vi "SIM Runge-Kutta (array).vi"(3 "Simulation data":T1={"continuous integrator"=enum."RK 1 (Euler)", "initial time"=0.1, "final time"=4.0, "step size"=600.0, "proposed step size"=1e-07, "max step size"=0.001, "min step size"=0.0, "discrete time step"=0.0, "max step ratio"=3.0, "Diag Eval Stage"=enum."Major Substep", "Substep Index"=0, "Timestep Index"=10.0, "simulation time"=0.0, "current timestep base"=0.01, "proposed step time"=0.0, "absolute tolerance"=0.0, "relative tolerance"=0.0, "step accepted?"=FALSE, "step complete?"=FALSE, "Halt?"=FALSE, "reset integrator?"=FALSE, "machine epsilon"=6.0, "min float"=0.0, "error"={"status"=FALSE, "code"=0, "source"=""}, "Method Order"=0, "Finished Late [i-1]"=FALSE, "Discrete step?"=FALSE, "NaN and Inf check?"=FALSE, "Final Timestep Index"=0.0, "(maj+disc)or(init)?"=FALSE, "Full Solver Reset"=TRUE, "Execution Mode"=enum."Simulate to Completion", "check vector sizes?"=FALSE, "solver handles zc?"=FALSE, "Simulation Registry"={"Current Idx"=0, "Node Tags"=[], "Node Headers"=[], "Node Data"=[], "Cont State data"={"inputs"=[], "outputs"=[], "reset"=[], "lower limits"=[], "upper limits"=[], "limit types"=[], "reset types"=[], "initial conditions"=[], "reset I.C."=[], "limited?"=[], "State Names"=[]}, "DiscreteInfo"={"tick period (sec)"=0.0, "time (ticks)"=0, "fire?"=[], "registry"={"period (sec)"=[], "skew (sec)"=[], "period (tick)"=[], "skew (tick)"=[]}, "discrete \nblocks?"=FALSE, "steps per tick"=0.0, "steps to tick"=0.0, "discrete \ntick?"=FALSE}, "Disc State data"={"Disc States"=[], "State Names"=[]}, "Registry Error"={"Error Block ID"=0, "code"=0}, "ZC Indices"=[]}, "variable step solver?"=FALSE, "First Substep?"=FALSE, "Continuous States?"=FALSE} {"min float" format="%.1e"; "proposed step size" format="%.1e"; "proposed step time" format="%.1e"; "max step ratio" format="%.1e"; "min step size" format="%.1e"; "machine epsilon" format="%.1e"; "discrete time step" format="%.1e"; "max step size" format="%.1e"; "current timestep base" format="%.1e"; "final time" format="%.1e"; "simulation time" format="%.1e"; "relative tolerance" format="%.1e"; "absolute tolerance" format="%.1e"; "Substep Index" format="%.1e"; "step size" format="%.1e"; "initial time" format="%.1e"}) -> (1 "Simulation data out":T1={"continuous integrator"=enum."RK 1 (Euler)", "initial time"=0.1, "final time"=4.0, "step size"=600.0, "proposed step size"=1e-07, "max step size"=0.001, "min step size"=0.0, "discrete time step"=0.0, "max step ratio"=3.0, "Diag Eval Stage"=enum."Major Substep", "Substep Index"=0, "Timestep Index"=10.0, "simulation time"=0.0, "current timestep base"=0.01, "proposed step time"=0.0, "absolute tolerance"=0.0, "relative tolerance"=0.0, "step accepted?"=FALSE, "step complete?"=FALSE, "Halt?"=FALSE, "reset integrator?"=FALSE, "machine epsilon"=6.0, "min float"=0.0, "error"={"status"=FALSE, "code"=0, "source"=""}, "Method Order"=0, "Finished Late [i-1]"=FALSE, "Discrete step?"=FALSE, "NaN and Inf check?"=FALSE, "Final Timestep Index"=0.0, "(maj+disc)or(init)?"=FALSE, "Full Solver Reset"=TRUE, "Execution Mode"=enum."Simulate to Completion", "check vector sizes?"=FALSE, "solver handles zc?"=FALSE, "Simulation Registry"={"Current Idx"=0, "Node Tags"=[], "Node Headers"=[], "Node Data"=[], "Cont State data"={"inputs"=[], "outputs"=[], "reset"=[], "lower limits"=[], "upper limits"=[], "limit types"=[], "reset types"=[], "initial conditions"=[], "reset I.C."=[], "limited?"=[], "State Names"=[]}, "DiscreteInfo"={"tick period (sec)"=0.0, "time (ticks)"=0, "fire?"=[], "registry"={"period (sec)"=[], "skew (sec)"=[], "period (tick)"=[], "skew (tick)"=[]}, "discrete \nblocks?"=FALSE, "steps per tick"=0.0, "steps to tick"=0.0, "discrete \ntick?"=FALSE}, "Disc State data"={"Disc States"=[], "State Names"=[]}, "Registry Error"={"Error Block ID"=0, "code"=0}, "ZC Indices"=[]}, "variable step solver?"=FALSE, "First Substep?"=FALSE, "Continuous States?"=FALSE} {"min float" format="%.1e"; "proposed step size" format="%.1e"; "proposed step time" format="%.1e"; "max step ratio" format="%.1e"; "min step size" format="%.1e"; "machine epsilon" format="%.1e"; "discrete time step" format="%.1e"; "max step size" format="%.1e"; "current timestep base" format="%.1e"; "final time" format="%.1e"; "simulation time" format="%.1e"; "relative tolerance" format="%.1e"; "absolute tolerance" format="%.1e"; "Substep Index" format="%.1e"; "step size" format="%.1e"; "initial time" format="%.1e"})   [LabVIEW 2014]
uses:
  SIM simulation data.ctl
  SIM integration method.ctl
  SIM diagram eval stage.ctl
  SIMSCR Execution Mode.ctl
  SIM Simulation Registry.ctl
  SIM Registry Node Header.ctl
  SIM Registry Node Record.ctl
  SIM trigger type.ctl
  SIM solver state data.ctl
  SIM limit type.ctl
  SIM discrete data.ctl
  SIM Discrete state data.ctl
  SIM Simulation Registry Error.ctl
  SIM limit signal (array).vi
panel:
  # "General Runge-Kutta integrator of order s.\n\nSolves the initial value problem \n\ny'(t) = f(t,y)\n\nby propogating the solution from y(t_n) to y(t_(n+1)), using the intermediate function evaluations k_i. The stepsize is defined as h = t_(n+1) - t_n.\n\nk_i = f( t_n + c_i h, y_n + h sum(j = 1 to s)(a_ij k_j) ) (1 <= i <= s)\n\ny_(n+1) = y_n + h sum(j = 1 to s)(a_(s-1)j k_j )\n\nNOTE This VI is paired with a time advancer that makes the simulation time appropriate for evaluating the k_i.\n\nNOTE This implementation assumes that c_0 = 0 and that\na_0j = 0 for a <= j <= s. The first row (all zeros) of the matrix a\nis omitted, and the last row of a stores the coefficients for the final output. Consequently, in the equation for k_i, a_ij should really read a_(i-1)j ."
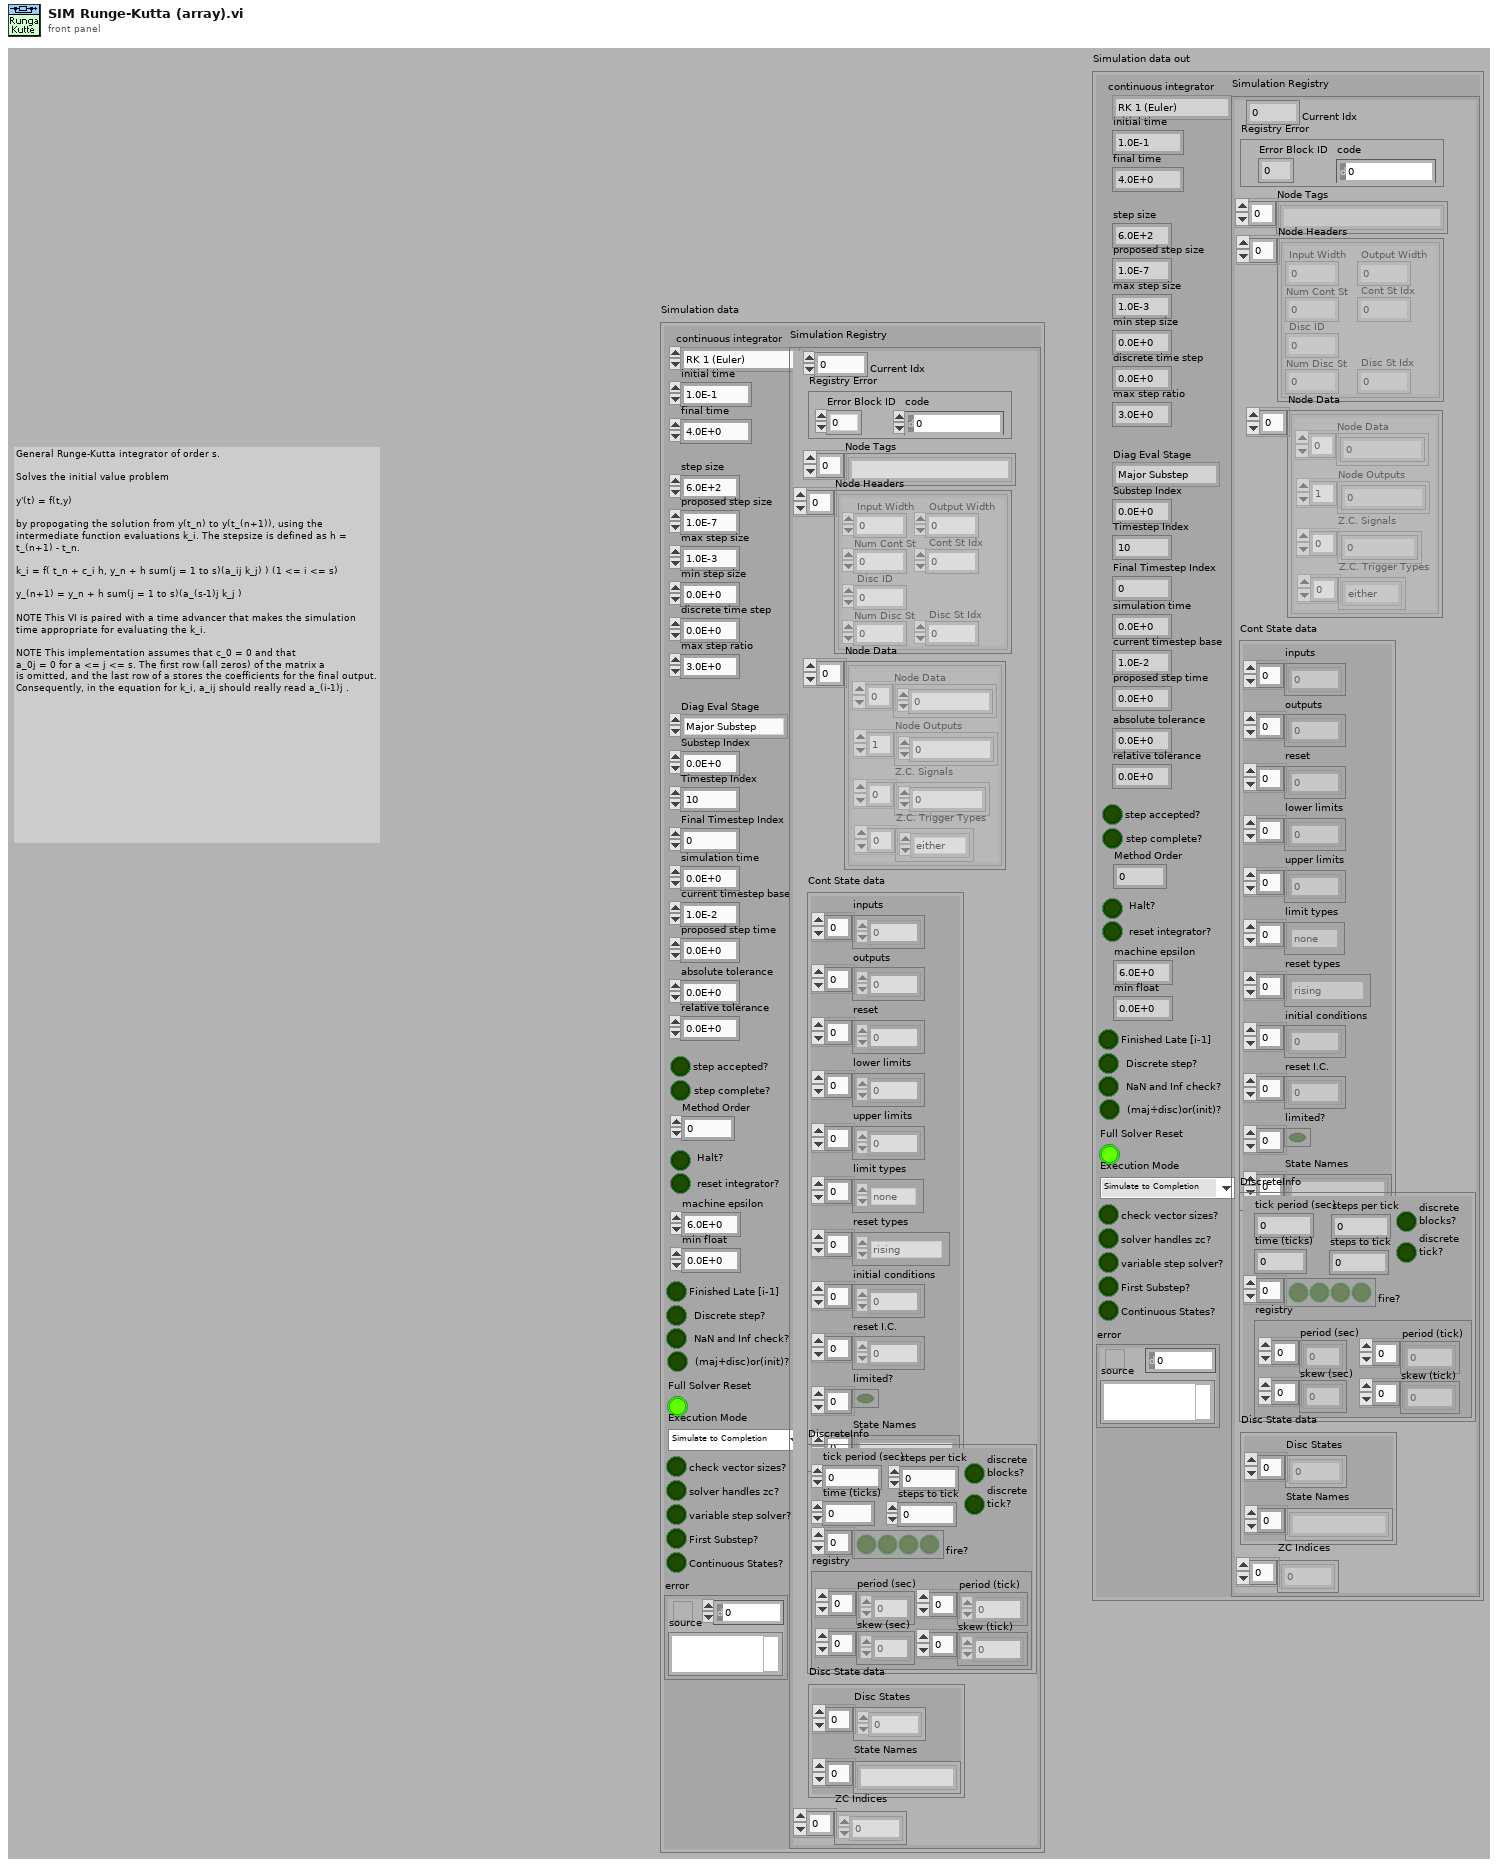
[diagram p1: front panel]
types:
  T1 = typedef "SIM simulation data.ctl" = cluster{"continuous integrator":T2, "initial time":dbl, "final time":dbl, "step size":dbl, "proposed step size":dbl, "max step size":dbl, "min step size":dbl, "discrete time step":dbl, "max step ratio":dbl, "Diag Eval Stage":T3, "Substep Index":i32, "Timestep Index":dbl, "simulation time":dbl, "current timestep base":dbl, "proposed step time":dbl, "absolute tolerance":dbl, "relative tolerance":dbl, "step accepted?":bool, "step complete?":bool, "Halt?":bool, "reset integrator?":bool, "machine epsilon":dbl, "min float":dbl, "error":errorcluster, "Method Order":u32, "Finished Late [i-1]":bool, "Discrete step?":bool, "NaN and Inf check?":bool, "Final Timestep Index":dbl, "(maj+disc)or(init)?":bool, "Full Solver Reset":bool, "Execution Mode":T4, "check vector sizes?":bool, "solver handles zc?":bool, "Simulation Registry":T5, "variable step solver?":bool, "First Substep?":bool, "Continuous States?":bool}
  T2 = typedef "SIM integration method.ctl" = enum16{"RK 1 (Euler)", "Linearizer", "State Query", "Trim Eval", "Adams", "RK 3", "RK 4", "RK 45", "BDF", "RK 2", "RK 23", "Rosenbrock", "Discrete States Only"}
  T3 = typedef "SIM diagram eval stage.ctl" = enum16{"Init", "Minor Substep", "Major Substep", "Final"}
  T4 = typedef "SIMSCR Execution Mode.ctl" = enum16{"Simulate to Completion", "Single Time-Step Simulation (Fixed Step Only)"}
  T5 = typedef "SIM Simulation Registry.ctl" = cluster{"Current Idx":i32, "Node Tags":string[], "Node Headers":T6[], "Node Data":T7[], "Cont State data":T9, "DiscreteInfo":T11, "Disc State data":T12, "Registry Error":T13, "ZC Indices":i32[]}
  T6 = typedef "SIM Registry Node Header.ctl" = cluster{"Input Width":i32, "Disc ID":i32, "Num Cont St":i32, "Cont St Idx":i32, "Num Disc St":i32, "Disc St Idx":i32, "Output Width":i32}
  T7 = typedef "SIM Registry Node Record.ctl" = cluster{"Node Data":dbl[], "Node Outputs":dbl[], "Z.C. Signals":dbl[], "Z.C. Trigger Types":T8[]}
  T8 = typedef "SIM trigger type.ctl" = enum16{"rising", "falling", "either", "none"}
  T9 = typedef "SIM solver state data.ctl" = cluster{"inputs":dbl[], "outputs":dbl[], "reset":dbl[], "lower limits":dbl[], "upper limits":dbl[], "limit types":T10[], "reset types":T8[], "initial conditions":dbl[], "reset I.C.":dbl[], "limited?":bool[], "State Names":string[]}
  T10 = typedef "SIM limit type.ctl" = enum16{"upper", "lower", "both", "none"}
  T11 = typedef "SIM discrete data.ctl" = cluster{"tick period (sec)":dbl, "time (ticks)":i32, "fire?":bool[], "registry":cluster{"period (sec)":dbl[], "skew (sec)":dbl[], "period (tick)":i32[], "skew (tick)":i32[]}, "discrete \nblocks?":bool, "steps per tick":dbl, "steps to tick":dbl, "discrete \ntick?":bool}
  T12 = typedef "SIM Discrete state data.ctl" = cluster{"Disc States":dbl[], "State Names":string[]}
  T13 = typedef "SIM Simulation Registry Error.ctl" = cluster{"Error Block ID":i32, "code":i32}
  T14 = typedef "SIM Runga-Kutte data - fixed step.ctl" = cluster{"weighting coefficients":dbl[][], "time step fractions":dbl[], "Number of sub steps":i32}
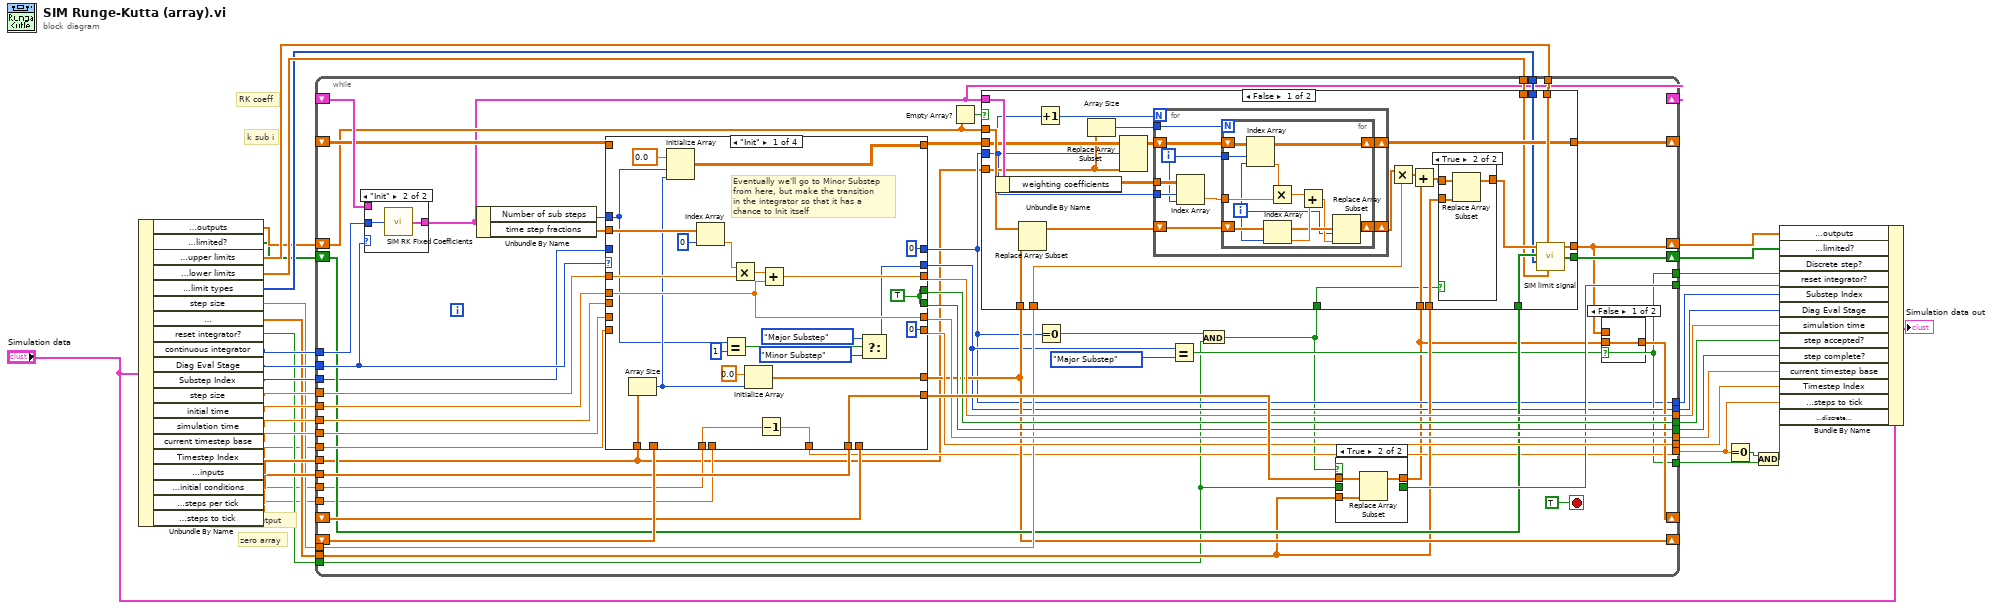
[diagram p0: block diagram]
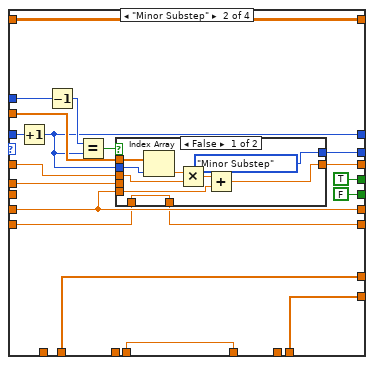
[diagram p6: hidden frame]
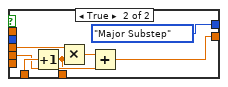
[diagram p7: hidden frame]
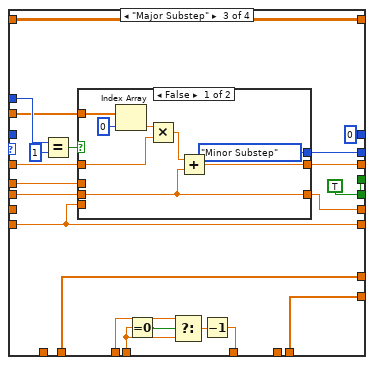
[diagram p8: hidden frame]
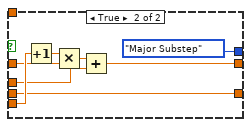
[diagram p9: hidden frame]
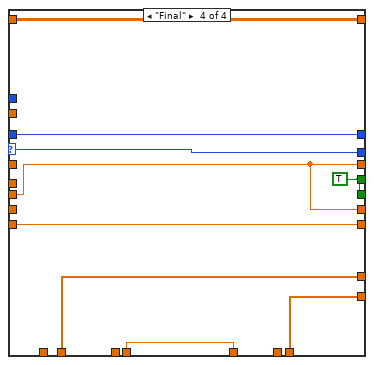
[diagram p10: hidden frame]
diagram:
  # "RK coeff"
  # "last major output"
  # "k sub i"
  # "zero array"
  n1 = Unbundle By Name("Simulation data") -> ("Simulation Registry.Cont State data.outputs"=w12:dbl[], "Simulation Registry.Cont State data.limited?"=w11:bool[], "Simulation Registry.Cont State data.upper limits"=w25:dbl[], "Simulation Registry.Cont State data.lower limits"=w24:dbl[], "Simulation Registry.Cont State data.limit types"=w23:T10[], "step size"=w16:dbl, "Simulation Registry.Cont State data.reset I.C."=w15:dbl[], "reset integrator?"=w13:bool, "continuous integrator"=w35:T2, "Diag Eval Stage"=w34:T3, "Substep Index"=w33:i32, "step size"=w32:dbl, "initial time"=w31:dbl, "simulation time"=w30:dbl, "current timestep base"=w29:dbl, "Timestep Index"=w9:dbl, "Simulation Registry.Cont State data.inputs"=w28:dbl[], "Simulation Registry.Cont State data.initial conditions"=w27:dbl[], "Simulation Registry.DiscreteInfo.steps per tick"=w6:dbl, "Simulation Registry.DiscreteInfo.steps to tick"=w5:dbl)
  n2 = while {
    shift-right: [w60] -> _
    shift-left: _ -> [w84]
    tunnel: w23 -> [w48]
    tunnel: w24 -> [w58]
    tunnel: w25 -> [w63]
    shift-right: [w55] -> _
    shift-left: _ -> [w81]
    shift-right: [w59] -> _
    shift-left: _ -> [w83]
    tunnel: [w49] -> w8
    shift-right: [w38] -> _
    shift-left: _ -> [w87]
    tunnel: w35 -> [w78]
    tunnel: w34 -> [w77]
    tunnel: w33 -> [w51]
    tunnel: w32 -> [w76]
    tunnel: w31 -> [w75]
    tunnel: w30 -> [w74]
    tunnel: w29 -> [w73]
    tunnel: w9 -> [w72]
    tunnel: w28 -> [w44]
    tunnel: w27 -> [w71]
    tunnel: [w47] -> w22
    tunnel: [w50] -> w21
    tunnel: [w70] -> w20
    tunnel: [w69] -> w19
    tunnel: [w68] -> w18
    tunnel: [w67] -> w17
    tunnel: [w66] -> w7
    tunnel: w16 -> [w65]
    tunnel: w15 -> [w57]
    tunnel: w13 -> [w42]
    tunnel: [w64] -> w14
    shift-right: [w56] -> w37
    shift-left: w12 -> [w40]
    shift-right: [w62] -> w10
    shift-left: w11 -> [w61]
    tunnel: w6 -> [w53]
    tunnel: w5 -> [w54]
    tunnel: [w52] -> w4
    tunnel: [w49] -> w2
    stop <- TRUE stop-if-true
    n3 = case shown="\"Init\"" w77 {
      tunnel: [w253 w255] -> w38
      tunnel: w87 -> [w253 _]
      tunnel: w78 -> [_ w254]
      frame Default {
      }
      frame "Init" {
        n4 = call "SIM RK Fixed Coefficients.vi"("continuous integrator"=w254) -> ("Runga-Kutte data out"=w255:T14)
      }
    }
    n5 = Unbundle By Name(w38) -> ("Number of sub steps"=w86:i32, "time step fractions"=w85:dbl[])
    n6 = case shown="\"Init\"" w77 {
      selector: w77 -> [_ _ _ w250]
      tunnel: w76 -> [w168 w183 w225 _]
      tunnel: [w165 w188 w223 w249] -> w67
      tunnel: w73 -> [_ w188 _ _]
      tunnel: w85 -> [w171 w190 w219 _]
      tunnel: [w166 w189 w220 w249] -> w70
      tunnel: w72 -> [_ w174 w213 w247]
      tunnel: w86 -> [w149 w187 w227 _]
      tunnel: [w152 w180 w217 w250] -> w50
      tunnel: w75 -> [w165 w179 w224 _]
      tunnel: [0 ("Timestep Index") w173 w213 w247] -> w66
      tunnel: w74 -> [_ _ w221 w249]
      tunnel: [w150 TRUE w207 w248] -> w69
      tunnel: [w150 FALSE w207 w248] -> w68
      tunnel: w51 -> [_ w182 _ w252]
      tunnel: [0 w178 0 ("Substep Index") w252] -> w47
      tunnel: w44 -> [w162 _ _ _]
      tunnel: [w158 w176 w216 w251] -> w46
      tunnel: w84 -> [_ w176 w216 w251]
      tunnel: [w157 w177 w215 w245] -> w59
      tunnel: w83 -> [_ w177 w215 w245]
      tunnel: w81 -> [_ w175 w214 w246]
      tunnel: [w151 w175 w214 w246] -> w80
      tunnel: w71 -> [w151 _ _ _]
      tunnel: w54 -> [_ w172 w209 w244]
      tunnel: w53 -> [w147 _ w210 _]
      tunnel: [w148 w172 w208 w244] -> w52
      frame "Init" {
        w150 = TRUE
        # "Eventually we'll go to Minor Substep from here, but make the transition in the integrator so that it has a chance to Init itself"
        n7 = Array Size(array=w162) -> (size(s)=w159:i32)
        n8 = Initialize Array(0.0 ("element"), w149, w159) -> (w158:dbl[][])
        n9 = Index Array(array=w171, index=0) -> (element=w169:dbl)
        n10 = Equal?(x=w149, y=1) -> (x = y?=w153:bool)
        n11 = Multiply(x=w169, y=w168) -> (x*y=w167:dbl)
        n12 = Initialize Array(0.0 ("element"), w159) -> (w157:dbl[])
        n13 = Decrement(x=w147) -> (x-1=w148:dbl)
        n14 = Add(x=w167, y=w165) -> (x+y=w166:dbl)
        n15 = Select(t=SIM_diagram_eval_stage."Major Substep", s=w153, f=SIM_diagram_eval_stage."Minor Substep" ("Diagram Eval Stage")) -> (s? t:f=w152:T3)
      }
      frame "Minor Substep" {
        n16 = Increment(x=w182) -> (x+1=w178:i32)
        n17 = Decrement(x=w187) -> (x-1=w186:i32)
        n18 = Equal?(x=w186, y=w178) -> (x = y?=w181:bool)
        n19 = case shown="False" w181 {
          tunnel: w190 -> [w199 _]
          tunnel: [w196 w201] -> w189
          tunnel: w188 -> [w195 _]
          tunnel: w183 -> [w194 w204]
          tunnel: w178 -> [w193 _]
          tunnel: [SIM_diagram_eval_stage."Minor Substep" ("f") SIM_diagram_eval_stage."Major Substep" ("Diagram Eval Stage")] -> w180
          tunnel: w174 -> [w191 w205]
          tunnel: w179 -> [_ w202]
          tunnel: [w191 w200] -> w173
          frame False {
            n20 = Index Array(array=w199, index=w193) -> (element=w198:dbl)
            n21 = Multiply(x=w198, y=w194) -> (x*y=w197:dbl)
            n22 = Add(x=w197, y=w195) -> (x+y=w196:dbl)
          }
          frame True {
            n23 = Increment(x=w205) -> (x+1=w200:dbl)
            n24 = Multiply(x=w204, y=w200) -> (x*y=w203:dbl)
            n25 = Add(x=w203, y=w202) -> (x+y=w201:dbl)
          }
        }
      }
      frame "Major Substep" {
        w207 = TRUE
        n26 = Equal?(x=w227, y=1 ("x")) -> (x = y?=w222:bool)
        n27 = case shown="False" w222 {
          tunnel: w225 -> [w231 w240]
          tunnel: w213 -> [_ w242]
          tunnel: w224 -> [_ w239]
          tunnel: w221 -> [w228 w236]
          tunnel: [w228 w236] -> w223
          tunnel: [SIM_diagram_eval_stage."Minor Substep" SIM_diagram_eval_stage."Major Substep"] -> w217
          tunnel: [w229 w237] -> w220
          tunnel: w219 -> [w232 _]
          frame False {
            n28 = Index Array(array=w232, index=0) -> (element=w233:dbl)
            n29 = Multiply(x=w233, y=w231) -> (x*y=w230:dbl)
            n30 = Add(x=w230, y=w228) -> (x+y=w229:dbl)
          }
          frame True {
            n31 = Increment(x=w242) -> (x+1=w241:dbl)
            n32 = Multiply(x=w241, y=w240) -> (x*y=w238:dbl)
            n33 = Add(x=w238, y=w239) -> (x+y=w237:dbl)
          }
        }
        n34 = Equal To 0?(x=w209) -> (x = 0?=w212:bool)
        n35 = Select(t=w210, s=w212, f=w209) -> (s? t:f=w211:dbl)
        n36 = Decrement(x=w211) -> (x-1=w208:dbl)
      }
      frame "Final" {
        w248 = TRUE
      }
    }
    n37 = Empty Array?(array=w40) -> (empty?=w41:bool)
    n38 = Equal To 0?(x=w47) -> (x = 0?=w43:bool)
    n39 = Equal?(x=w50, y=SIM_diagram_eval_stage."Major Substep") -> (x = y?=w49:bool)
    n40 = And(x=w43, y=w42) -> (x .and. y?=w45:bool)
    n41 = case shown="True" w45 {
      tunnel: [w143 w146] -> w39
      tunnel: w80 -> [w143 w145]
      tunnel: w57 -> [_ w144]
      tunnel: [w142 _] -> w64
      tunnel: w42 -> [w142 _]
      frame False {
      }
      frame True {
        n42 = Replace Array Subset(array=w145, new element=w144) -> (w146:dbl[])  [unwired: 1 in]
      }
    }
    n43 = case shown="False" w41 {
      tunnel: w38 -> [w109 _]
      tunnel: w65 -> [w108 _]
      tunnel: w63 -> [w107 _]
      tunnel: [w106 w139] -> w62
      tunnel: w61 -> [w105 w139]
      tunnel: [w104 w137] -> w60
      tunnel: w40 -> [w103 w138]
      tunnel: w59 -> [w102 _]
      tunnel: w58 -> [w99 _]
      tunnel: w57 -> [w98 _]
      tunnel: [w97 w138] -> w56
      tunnel: w39 -> [w96 _]
      tunnel: w48 -> [w93 _]
      tunnel: w47 -> [w88 _]
      tunnel: w46 -> [w92 w137]
      tunnel: w45 -> [w95 _]
      tunnel: w44 -> [w90 _]
      frame False {
        n44 = Unbundle By Name(w109) -> ("weighting coefficients"=w89:dbl[][])
        n45 = Replace Array Subset(array=w103, new element=w102) -> (w101:dbl[])  [unwired: 1 in]
        n46 = Increment(x=w88) -> (x+1=w110:i32)
        n47 = Array Size(array=w90) -> (size(s)=w94:i32)
        n48 = Replace Array Subset(array=w92, new element=w90, index (row)=w88) -> (w91:dbl[][])  [unwired: 1 in]
        n49 = for {
          N: w110 -> [_]
          shift-right: [w125] -> w112
          shift-left: w101 -> [w126]
          shift-right: [w124] -> w104
          shift-left: w91 -> [w122]
          tunnel: w94 -> [w123]
          tunnel: w89 -> [w121]
          tunnel: w88 -> [w120]
          i -> [w119]
          n50 = Index Array(array=w121, index (row)=w120, index (col)=w119) -> (element=w118:dbl)
          n51 = for {
            N: w123 -> [_]
            tunnel: w118 -> [w136]
            shift-right: [w131] -> w125
            shift-left: w126 -> [w133]
            shift-right: [w127] -> w124
            shift-left: w122 -> [w127]
            tunnel: w119 -> [w130]
            i -> [w129]
            n52 = Index Array(array=w127, index (row)=w130, index (col)=w129) -> (element=w128:dbl)
            n53 = Index Array(array=w133, index=w129) -> (element=w134:dbl)
            n54 = Multiply(x=w128, y=w136) -> (x*y=w135:dbl)
            n55 = Add(x=w135, y=w134) -> (x+y=w132:dbl)
            n56 = Replace Array Subset(array=w133, new element=w132, index=w129) -> (w131:dbl[])
          }
        }
        n57 = Multiply(x=w112, y=w108) -> (x*y=w111:dbl[])
        n58 = Add(x=w111, y=w96) -> (x+y=w100:dbl[])
        n59 = case shown="True" w95 {
          tunnel: [w114 w116] -> w113
          tunnel: w100 -> [w114 w117]
          tunnel: w98 -> [_ w115]
          frame False {
          }
          frame True {
            n60 = Replace Array Subset(array=w117, new element=w115) -> (w116:dbl[])  [unwired: 1 in]
          }
        }
        n61 = call-poly "SIM limit signal.vi"("lower limits"=w99, "upper limits"=w107, "limit types"=w93, "limited? in"=w105, "inputs"=w113) -> ("limited? out"=w106:bool[], "outputs"=w97:dbl[])  [unwired: 1 in, 4 out]
      }
      frame True {
      }
    }
    n62 = case shown="False" w49 {
      tunnel: [w140 w141] -> w55
      tunnel: w56 -> [_ w141]
      tunnel: w39 -> [w140 _]
      frame False {
      }
      frame True {
      }
    }
  }
  n63 = Equal To 0?(x=w4) -> (x = 0?=w3:bool)
  n64 = And(x=w3, y=w2) -> (x .and. y?=w1:bool)
  n65 = Bundle By Name(cluster="Simulation data", "Simulation Registry.Cont State data.outputs"=w37, "Simulation Registry.Cont State data.limited?"=w10, "Discrete step?"=w8, "reset integrator?"=w14, "Substep Index"=w22, "Diag Eval Stage"=w21, "simulation time"=w20, "step accepted?"=w19, "step complete?"=w18, "current timestep base"=w17, "Timestep Index"=w7, "Simulation Registry.DiscreteInfo.steps to tick"=w4, "Simulation Registry.DiscreteInfo.discrete \ntick?"=w1) -> (→"Simulation data out":T1)
